vi "CallWeb.vi"(4 "Longitud":string="-66.88\n", 5 "Latitud":string="10.41", 6 "Fecha final":timestamp format="%<%Y/%m/%d>T", 7 "Fecha inicial":timestamp format="%<%Y/%m/%d>T") -> (0 "error?":bool, 1 "fecha":dbl[](array[numeric]), 2 "temperatura":dbl[](array[numeric]), 3 "irradiancia":dbl[](array[numeric]))   [LabVIEW 2014]
uses:
  <vilib>/addons/database/Auxilliary.llb/DB Tools Format Datetime String (Time Stamp).vi
  <vilib>/httpClient/LabVIEWHTTPClient.lvlib
  <vilib>/addons/database/NI_Database_API.lvlib
panel:
  out "message":string=" INSTRUCTIONS:\r\rNormal Use:  When using subVIs that incorporate the error in/error out (or error I/O) structure, place this handler where you want to inform the user of an error, typically at the end of the I/O data path, as the last action of the program.  If the error in error? is ERROR, the handler creates a message describing the error and its source.  If the type of dialog = 1 (default), the message is displayed to the user, who can only acknowedge it.  If the type = 2, the user can acknowledge the message or abort execution; aborting a program with active I/O is not recommended.  If the type = 0, no message is displayed; this is used to process the error programmatically, and the error out cluster elements are wired to individual terminals for that reason.  \r\rOther Use:\n\r\nlocal testing.  To test the error code of a subVI or function that does not have the error I/O structure, you can wire its error code and a source string to the local error code and error source inputs.  If error in error? indicates no error and error code is not equal to 0, the local code and source are substituted for the error in values, and error? is set TRUE (ERROR)."
  out "result string":string
  in  "Año":dbl
  in  "Mes":dbl
  in  "Dia":dbl
  out "Irradancia":dbl
  out "Temperatura":dbl
  out "body":string
  out "headers":string
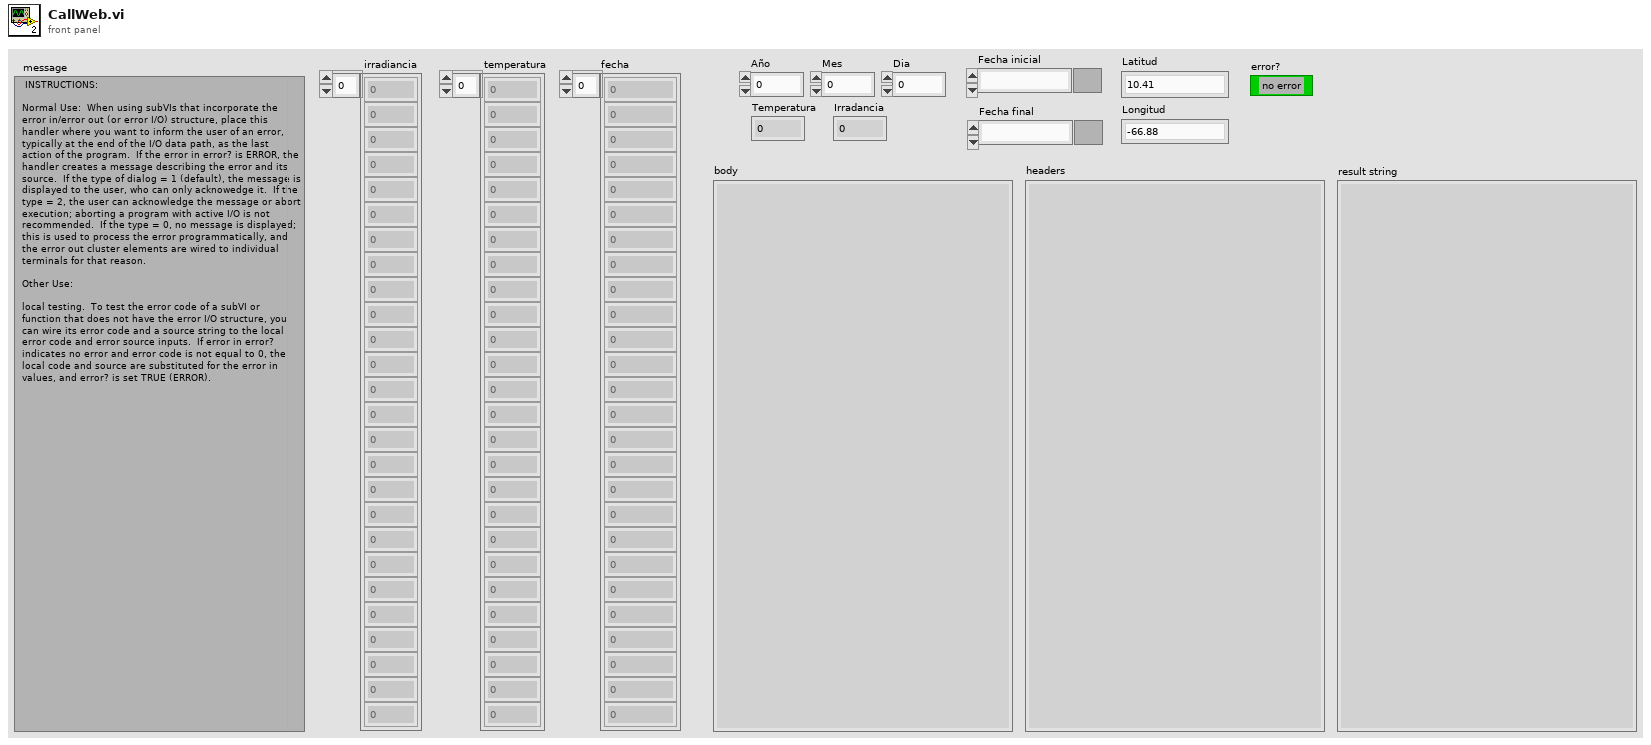
[diagram p1: front panel]
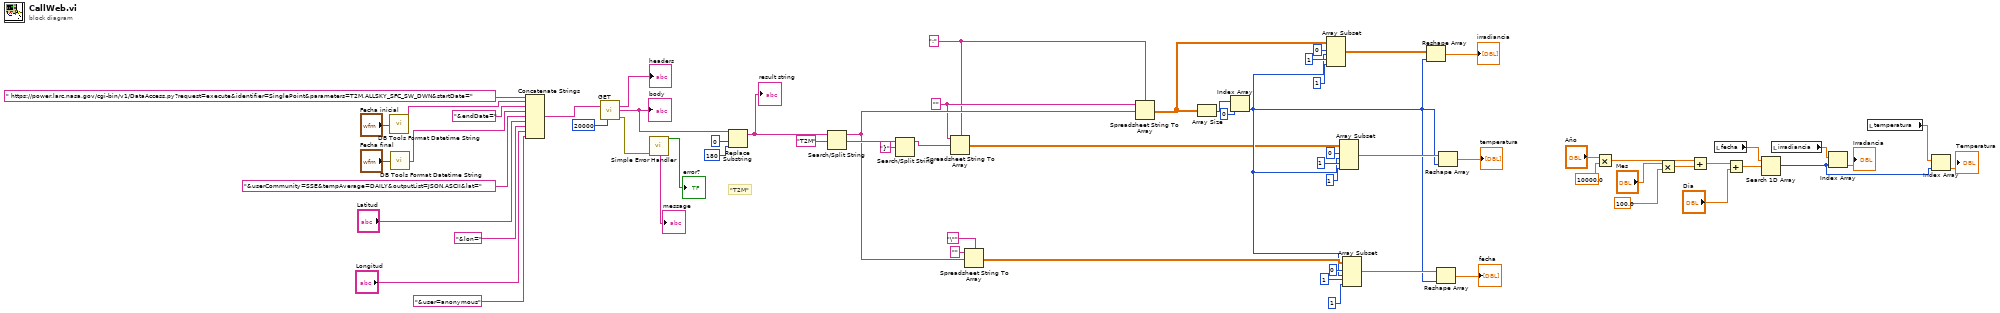
[diagram p0: block diagram]
diagram:
  w19 = ":"
  w20 = ""
  # "\"T2M\""
  n1 = call-poly <vilib>:"DB Tools Format Datetime String.vi"("time stamp"="Fecha inicial") -> ("date/time string"=w8:string)
  n2 = call-poly <vilib>:"DB Tools Format Datetime String.vi"("time stamp"="Fecha final") -> ("date/time string"=w14:string)
  n3 = Concatenate Strings(" https://power.larc.nasa.gov/cgi-bin/v1/DataAccess.py?request=execute&identifier=SinglePoint&parameters=T2M,ALLSKY_SFC_SW_DWN&startDate=", w8, "&endDate=", w14, "&userCommunity=SSE&tempAverage=DAILY&outputList=JSON,ASCII&lat=" ("url"), "Latitud", "&lon=" ("url"), "Longitud", "&user=anonymous" ("url")) -> (w11:string)
  n4 = call <vilib>:"GET.vi"("url"=w11, "timeout (10000)"=20000) -> ("headers"=→"headers":string, "body"=w3:string, "error out"=w6:errorcluster)  [unwired: 10 in, 1 out]
  "body" <- w3
  n5 = call <vilib>:"Simple Error Handler.vi"("error in (no error)"=w6) -> ("error?"=→"error?":bool, "message"=→"message":string)  [unwired: 4 in, 3 out]
  n6 = Replace Substring(2:180 ("length (len. of substring)"), 3:0 ("length (len. of substring)"), 5:w3) -> (1:w63:string)  [unwired: 1 in, 1 out]
  "result string" <- w63
  n7 = Search/Split String(string=w63, search string/char (-)="T2M") -> (substring before match=w57:string, match + rest of string=w62:string)  [unwired: 1 in, 1 out]
  n8 = Search/Split String(string=w62, search string/char (-)="}") -> (substring before match=w60:string)  [unwired: 1 in, 2 out]
  n9 = Spreadsheet String To Array(delimiter (Tab)=w19, format string=w20, spreadsheet string=w60) -> (array=w36:dbl[][])  [unwired: 1 in]
  n10 = Spreadsheet String To Array(delimiter (Tab)="\"", format string="", spreadsheet string=w57) -> (array=w38:dbl[][])  [unwired: 1 in]
  n11 = Spreadsheet String To Array(delimiter (Tab)=w19, format string=w20, spreadsheet string=w57) -> (array=w51:dbl[][])  [unwired: 1 in]
  n12 = Array Size(array=w51) -> (size(s)=w56:i32[])
  n13 = Index Array(array=w56, index=0) -> (element=w37:i32)
  n14 = Array Subset "Array Subset"(array=w51, index (row)=0 ("index"), length (row)=w37, index (col)=1 ("index"), length (col)=1 ("length")) -> (w50:dbl[][])
  n15 = Array Subset "Array Subset"(array=w36, index (row)=0 ("index"), length (row)=w37, index (col)=1 ("index"), length (col)=1 ("length")) -> (w44:dbl[][])
  n16 = Array Subset "Array Subset"(array=w38, index (row)=0 ("index"), length (row)=w37, index (col)=1 ("index"), length (col)=1 ("length")) -> (w39:dbl[][])
  n17 = Reshape Array(w50, w37) -> (→"irradiancia":dbl[])
  n18 = Reshape Array(w39, w37) -> (→"fecha":dbl[])
  n19 = Reshape Array(w44, w37) -> (→"temperatura":dbl[])
  n20 = Multiply(x="Año", y=10000.0) -> (x*y=w33:dbl)
  n21 = Multiply(x="Mes", y=100.0) -> (x*y=w32:dbl)
  n22 = Add(x=w33, y=w32) -> (x+y=w31:dbl)
  n23 = local read "fecha"() -> (w26:dbl[])
  n24 = Add(x=w31, y="Dia") -> (x+y=w27:dbl)
  n25 = Search 1D Array(1D array=w26, element=w27) -> (index of element=w22:i32)  [unwired: 1 in]
  n26 = local read "irradiancia"() -> (w25:dbl[])
  n27 = Index Array(array=w25, index=w22) -> (element=→"Irradancia":dbl)
  n28 = local read "temperatura"() -> (w23:dbl[])
  n29 = Index Array(array=w23, index=w22) -> (element=→"Temperatura":dbl)
